vi "AlliGator Get Dataset Series Timestamp & Intensity Correction.vi"(6 "Current Data Set":i32, 7 "Time Step":dbl[unit], 8 "Use Intensity Correction":bool, 9 "Intensity Corrections":dbl[](array[numeric]), 10 "Use File Timestamp":bool, 11 "Dataset Series Timestamps":dbl[](array[numeric])) -> (1 "Intensity Correction":dbl, 3 "Time Stamp (s)":dbl)   [LabVIEW 2021, in "AlliGator Intensity Corrections.lvlib"]
doc: "Get dataset timestamp and intensity corrections (if available and requested) or use defaults instead."
uses:
  AlliGator Intensity Corrections.lvlib
panel:
  # "see the AlliGator License on the block diagram (Ctrl+E or Window:Show Block Diagram)"
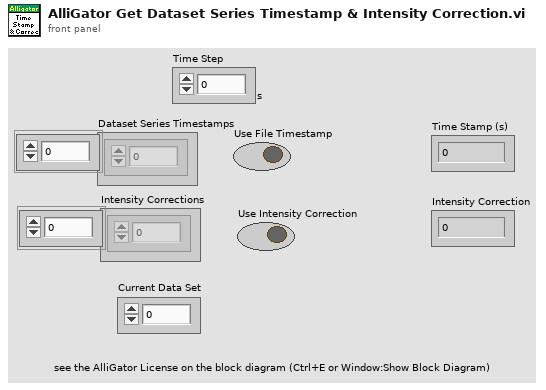
[diagram p1: front panel]
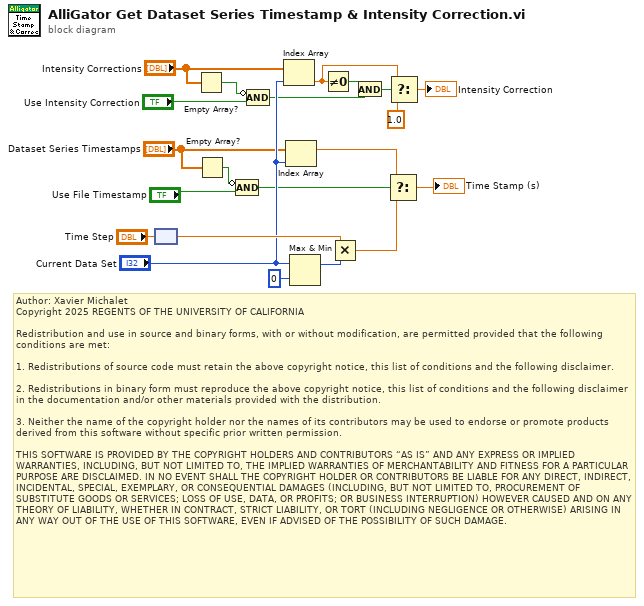
[diagram p0: block diagram]
diagram:
  # "Author: Xavier Michalet\nCopyright 2025 REGENTS OF THE UNIVERSITY OF CALIFORNIA\n\nRedistribution and use in source and binary forms, with or without modification, are permitted provided that the following conditions are met:\n\n1. Redistributions of source code must retain the above copyright notice, this list of conditions and the following disclaimer.\n\n2. Redistributions in binary form must reproduce the above copyright notice, this list of conditions and the following disclaimer in the documentation and/or other materials provided with the distribution.\n\n3. Neither the name of the copyright holder nor the names of its contributors may be used to endorse or promote products derived from this software without specific prior written permission.\n\nTHIS SOFTWARE IS PROVIDED BY THE COPYRIGHT HOLDERS AND CONTRIBUTORS “AS IS” AND ANY EXPRESS OR IMPLIED WARRANTIES, INCLUDING, BUT NOT LIMITED TO, THE IMPLIED WARRANTIES OF MERCHANTABILITY AND FITNESS FOR A PARTICULAR PURPOSE ARE DISCLAIMED. IN NO EVENT SHALL THE COPYRIGHT HOLDER OR CONTRIBUTORS BE LIABLE FOR ANY DIRECT, INDIRECT, INCIDENTAL, SPECIAL, EXEMPLARY, OR CONSEQUENTIAL DAMAGES (INCLUDING, BUT NOT LIMITED TO, PROCUREMENT OF SUBSTITUTE GOODS OR SERVICES; LOSS OF USE, DATA, OR PROFITS; OR BUSINESS INTERRUPTION) HOWEVER CAUSED AND ON ANY THEORY OF LIABILITY, WHETHER IN CONTRACT, STRICT LIABILITY, OR TORT (INCLUDING NEGLIGENCE OR OTHERWISE) ARISING IN ANY WAY OUT OF THE USE OF THIS SOFTWARE, EVEN IF ADVISED OF THE POSSIBILITY OF SUCH DAMAGE."
  n1 = node("Time Step") -> (w18:dbl)
  n2 = Empty Array?(array="Intensity Corrections") -> (empty?=w1:bool)
  n3 = Empty Array?(array="Dataset Series Timestamps") -> (empty?=w5:bool)
  n4 = Compound Arithmetic op=AND(invert w5, "Use File Timestamp") -> (w6:bool)
  n5 = Compound Arithmetic op=AND(invert w1, "Use Intensity Correction") -> (w2:bool)
  n6 = Index Array(array="Intensity Corrections", index="Current Data Set") -> (element=w11:dbl)
  n7 = Index Array(array="Dataset Series Timestamps", index="Current Data Set") -> (element=w16:dbl)
  n8 = Max & Min(x="Current Data Set", y=0) -> (max(x,y)=w9:i32)  [unwired: 1 out]
  n9 = Not Equal To 0?(x=w11) -> (x != 0?=w13:bool)
  n10 = Multiply(x=w18, y=w9) -> (x*y=w17:dbl)
  n11 = And(x=w13, y=w2) -> (x .and. y?=w12:bool)
  n12 = Select(t=w16, s=w6, f=w17) -> (s? t:f=→"Time Stamp (s)":dbl)
  n13 = Select(t=w11, s=w12, f=1.0) -> (s? t:f=→"Intensity Correction":dbl)
